vi "Load Cursors.vi"(0 "Display State In":T1, 5 "Path":path, 9 "Container State":T2, 11 "error in (no error)":errorcluster) -> (4 "Display State Out":T1, 15 "error out":errorcluster)   [LabVIEW 2014, in "Graph with cursors XControl.xctl"]
uses:
  Graph with cursors XControl.xctl
  <vilib>/_xctls/Container State.ctl
  Graph with cursors State.ctl
  <vilib>/_xctls/XControlSupport.lvlib
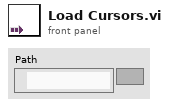
[diagram p1: front panel]
types:
  T1 = typedef "Graph with cursors XControl.xctl/Graph with cursors State.ctl" = cluster{"Cursor names":string[], "Cursor positions":dbl[], "Cursor pairs":i32, "Graph":refnum<vi>, "Prefix":string, "Base path":path}
  T2 = typedef "XControlSupport.lvlib/Container State.ctl" = cluster{"Indicator?":bool, "Run Mode?":bool, " Refnum":refnum<vi>}
  T3 = typedef "LVCursorListTypeDef.ctl" = cluster{"Name":string, "Color":u32, "Style":u8, "Point Style":u8, "Name Visible":bool, "Allow Drag":bool, "Cursor Mode":u32, "Plot":i32, "Index":i32, "Position":cluster{"X":dbl, "Y":dbl}, "X Scale":u32, "Y Scale":u32, "Watch Plots":i32[], "Watch All Plots":bool, "Plot Area":i32, "Label Offset":cluster{"X":dbl, "Y":dbl}}[]
  T4 = cluster{"Name":string, "Color":u32, "Style":u8, "Point Style":u8, "Name Visible":bool, "Allow Drag":bool, "Cursor Mode":u32, "Plot":i32, "Index":i32, "Position":cluster{"X":dbl, "Y":dbl}, "X Scale":u32, "Y Scale":u32, "Watch Plots":i32[], "Watch All Plots":bool, "Plot Area":i32, "Label Offset":cluster{"X":dbl, "Y":dbl}}
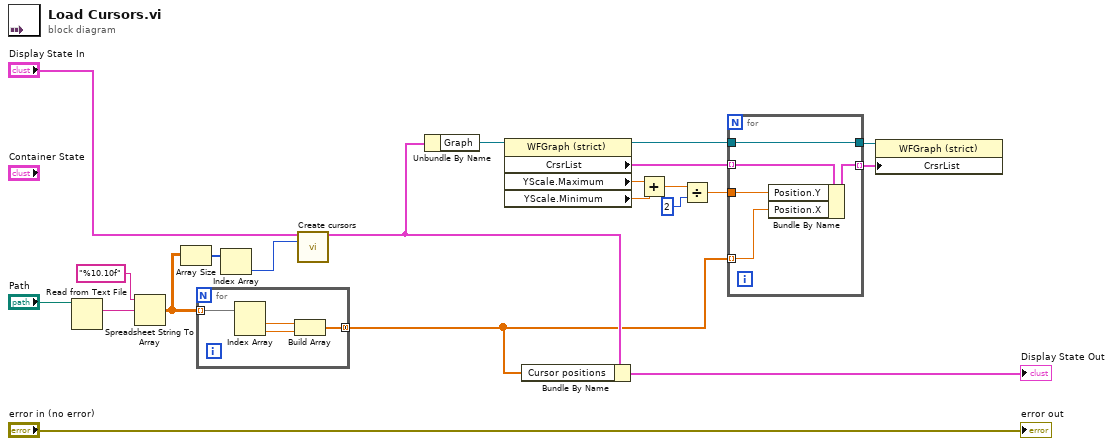
[diagram p0: block diagram]
diagram:
  n1 = Read from Text File(file (use dialog)="Path") -> (text=w9:string)  [unwired: 3 in, 3 out]
  n2 = Spreadsheet String To Array(format string="%10.10f", spreadsheet string=w9) -> (array=w7:dbl[][])  [unwired: 2 in]
  n3 = Array Size(array=w7) -> (size(s)=w6:i32[])
  n4 = for {
    tunnel: w7 -> [w25] mode=indexing
    tunnel: [w22] -> w3 mode=concatenating
    n5 = Index Array(array=w25) -> (element #1=w24:dbl, element #2=w23:dbl)  [unwired: 2 in]
    n6 = Build Array(w24, w23) -> (w22:dbl[])
  }
  n7 = Index Array(array=w6) -> (element=w1:i32)  [unwired: 1 in]
  n8 = call "Create cursors.vi"("Display State In"="Display State In", "Cursor pairs"=w1) -> ("Display State Out"=w4:T1)  [unwired: 12 in, 1 out]
  n9 = Unbundle By Name(w4) -> ("Graph"=w20:refnum<vi>)
  n10 = property class="WFGraph (strict)"(reference=w20) -> (reference out=w13:refnum<vi>, "CrsrList"=w14:T3, "YScale.Maximum"=w18:dbl, "YScale.Minimum"=w19:dbl)  [unwired: 1 in, 1 out]
  n11 = Bundle By Name(cluster=w4, "Cursor positions"=w3) -> (→"Display State Out":T1)
  n12 = Add(x=w18, y=w19) -> (x+y=w17:dbl)
  n13 = Divide(x=w17, y=u32 2) -> (x/y=w15:dbl)
  n14 = for {
    tunnel: w15 -> [w30]
    tunnel: w14 -> [w29] mode=indexing
    tunnel: [w28] -> w11 mode=indexing
    tunnel: [w27] -> w12
    tunnel: w13 -> [w27]
    tunnel: w3 -> [w26] mode=indexing
    n15 = Bundle By Name(cluster=w29, "Position.Y"=w30, "Position.X"=w26) -> (w28:T4)
  }
  n16 = property class="WFGraph (strict)"(reference=w12, "CrsrList"=w11) -> ()  [unwired: 1 in, 2 out]
  "error out" <- "error in (no error)"
